vi "itc_clearPixel.vi"   [LabVIEW 2016]
uses:
  <vilib>/rvi/DataTransferAndStorage/Container/XNode/niFpgaContainer.xnode
  <vilib>/eio/EIONode/EIONode.xnode
  <vilib>/rvi/FIFO/Fifo_Resource/nirvififoEmulationRead.vi
  <vilib>/rvi/eio/common/nirviEmuTemplateMethod_errors.vi
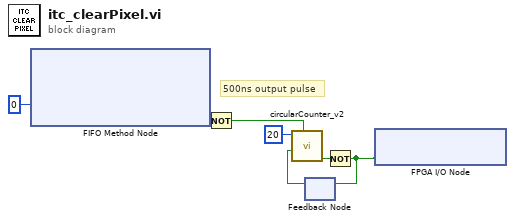
[diagram p0: block diagram]
diagram:
  # "500ns output pulse"
  n1 = xnode ("FIFO Method Node")("Timeout"=0) -> ("Timed Out?"=w5:bool)  [unwired: 1 in, 2 out]
  n2 = Not(x=w5) -> (.not. x?=w4:bool)
  n3 = feedback #1() -> (w2:bool)  [unwired: 1 in]
  n4 = call "circularCounter_v2.vi"("reset"=w4, "doStep"=w2, "maxCount"=u16 20) -> ("maxReached"=w3:bool)  [unwired: 5 in, 3 out]
  n5 = Not(x=w3) -> (.not. x?=w1:bool)
  n6 = feedback-in #1(w1) -> ()
  n7 = xnode "FPGA I/O Node"("itc-hdt.clearPixel"=w1) -> ()  [unwired: 1 in, 1 out]
